vi "Add Routing and Faulting Custom Device.vi"(8 "error in (no error)":errorcluster, 10 "Settings":T1, 11 "Target in":refnum<k24>) -> (0 "error out":errorcluster, 2 "RAF Custom Device":refnum<k24>, 3 "Target out":refnum<k24>)   [LabVIEW 2017, in "Switch Scripting.lvlib"]
uses:
  Switch Scripting.lvlib
  NationalInstruments.VeriStand.SystemDefinitionAPI
  Shared/Routing and Faulting Custom Device Settings.ctl
  Shared/Constants.vi
  Shared/Switch Shared.lvlib
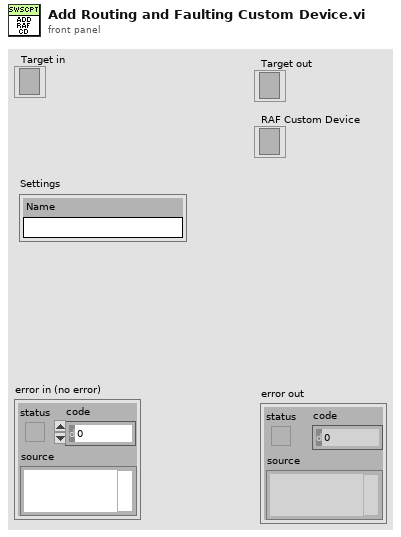
[diagram p1: front panel]
types:
  T1 = typedef "Switch Shared.lvlib/Routing and Faulting Custom Device Settings.ctl" = cluster{"Name":string}
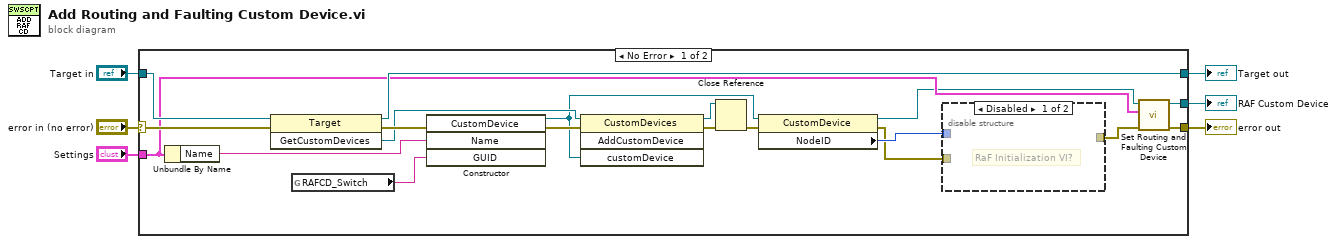
[diagram p0: block diagram]
diagram:
  n1 = case shown="No Error" "error in (no error)" {
    selector: "error in (no error)" -> [w25 w28]
    tunnel: [w16 w28] -> w6
    tunnel: "Target in" -> [w24 w27]
    tunnel: [w20 w27] -> w3
    tunnel: "Settings" -> [w14 _]
    tunnel: [w17 _] -> w1
    frame No Error {
      n2 = Unbundle By Name(w14) -> ("Name"=w15:string)
      n3 = invoke class="Target" method="GetCustomDevices"(reference=w24, error in=w25) -> (reference out=w20:refnum<k24>, error out=w23:errorcluster, "GetCustomDevices"=w22:refnum<k24>)  [unwired: 1 in]
      n4 = global read "Constants.vi" "RAFCD_Switch"() -> (w10:string)
      n5 = constructor class="CustomDevice"(error in=w23, "Name"=w15, "GUID"=w10) -> (reference out=w13:refnum<k24>, error out=w21:errorcluster)  [unwired: 2 in, 3 out]
      n6 = invoke class="CustomDevices" method="AddCustomDevice"(reference=w22, error in=w21, "customDevice"=w13) -> (reference out=w19:refnum<k24>, error out=w18:errorcluster)  [unwired: 1 in, 2 out]
      n7 = Close Reference(reference=w19, error in (no error)=w18) -> (error out=w11:errorcluster)
      n8 = property class="CustomDevice"(reference=w13, error in=w11) -> (reference out=w12:refnum<k24>, error out=w8:errorcluster, "NodeID"=w9:u64)
      n9 = disable-structure shown="Disabled" {
        disable-tunnel: w9 -> [_ _]
        disable-tunnel: w8 -> [_ w26]
        disable-tunnel: [_ w26] -> w7
        frame Disabled {
          # "RaF Initialization VI?"
        }
        frame Enabled {
        }
      }
      n10 = call "Set Routing and Faulting Custom Device.vi"("error in (no error)"=w7, "Settings"=w14, "RAF Custom Device in"=w12) -> ("error out"=w16:errorcluster, "RAF Custom Device out"=w17:refnum<k24>)  [unwired: 7 in]
    }
    frame Error {
    }
  }
  "Target out" <- w3
  "error out" <- w6
  "RAF Custom Device" <- w1
